vi "getStandaloneProgramStatus.vi"(0 "Pmx4exSaController in":refnum<class "Pmx4exSaController.lvclass">, 5 "error in (no error)":errorcluster) -> (14 "Pmx4exSaController out":refnum<class "Pmx4exSaController.lvclass">, 16 "status (out)":T1, 19 "error out":errorcluster)   [LabVIEW 2020, in "classes.lvlib" / "Pmx4exSaController.lvclass"]
doc: "Produced By:\n\n<B>Kod Integrations, LLC</B>\n4835 Marianne Drive\nMount Airy, MD 21771\nhttp://www.kodintegrations.com\nemail: info@kodintegrations.com\nphone: (240) 687-1288"
uses:
  Pmx4exSaController.lvclass
  C:/GEECS/Developers Version/source/Device Drivers/Newmark-NSC-A/Arcus Driver 3.0.0/ArcusUsbComm/classes/Controller/_Controller.lvclass
  common/controls/standalone_program_status.ctl
  Controller/_Controller.lvclass
  libraries/common.lvlib
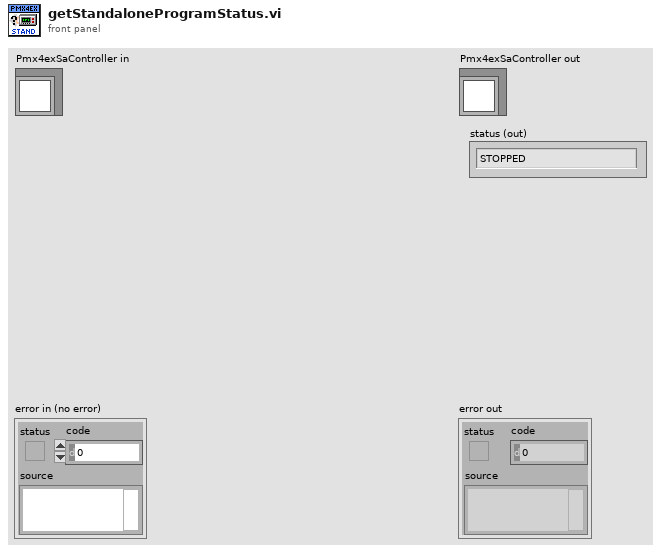
[diagram p1: front panel]
types:
  T1 = typedef "common.lvlib/standalone_program_status.ctl" = enum16{"STOPPED", "RUNNING", "PAUSED", "IN_ERROR"}
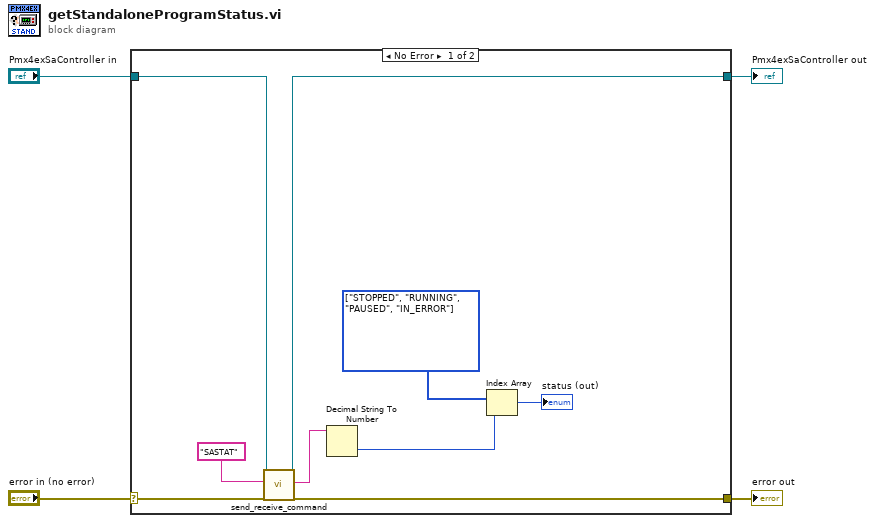
[diagram p0: block diagram]
diagram:
  n1 = case shown="No Error" "error in (no error)" {
    selector: "error in (no error)" -> [w13 w15]
    tunnel: [w12 w15] -> w3
    tunnel: [w10 w14] -> w1
    tunnel: "Pmx4exSaController in" -> [w11 w14]
    frame No Error {
      w6 = T1[] [enum."STOPPED", enum."RUNNING", enum."PAUSED", enum."IN_ERROR"] items=["STOPPED", "RUNNING", "PAUSED", "IN_ERROR"]
      n2 = call "send_receive_command.vi"("reference (in)"=w11, "ASCII Command (in)"="SASTAT", "error in (no error)"=w13) -> ("reference (out)"=w10:refnum<class "Pmx4exSaController.lvclass">, "response (out)"=w9:string, "error out"=w12:errorcluster)  [unwired: 12 in, 2 out]
      n3 = Decimal String To Number(string=w9) -> (number=w8:i32)  [unwired: 2 in, 1 out]
      n4 = Index Array(array=w6, index=w8) -> (element=→"status (out)":T1)
    }
    frame Error {
    }
  }
  "error out" <- w3
  "Pmx4exSaController out" <- w1
